vi "CRYOperator Message.vi"() -> ()   [LabVIEW 2013]
uses:
  SubVI/CRYMisc vis settings global.vi
panel:
  in  "sButton":string
  in  "sOperator Type":string
  in  "index":i32
  in  "StateOut":bool
  in  "Stop":bool
  in  "pVI":refnum<vi>
  in  "sMsgCommand":string="REMOTE_COMMAND"
  # "Operator Message Processing."
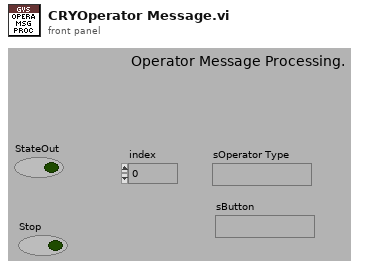
[diagram p1: front panel]
types:
  T1 = cluster{"VI Ref":refnum<vi>[], "VI nID":i32[], "Title nID":i32[]}
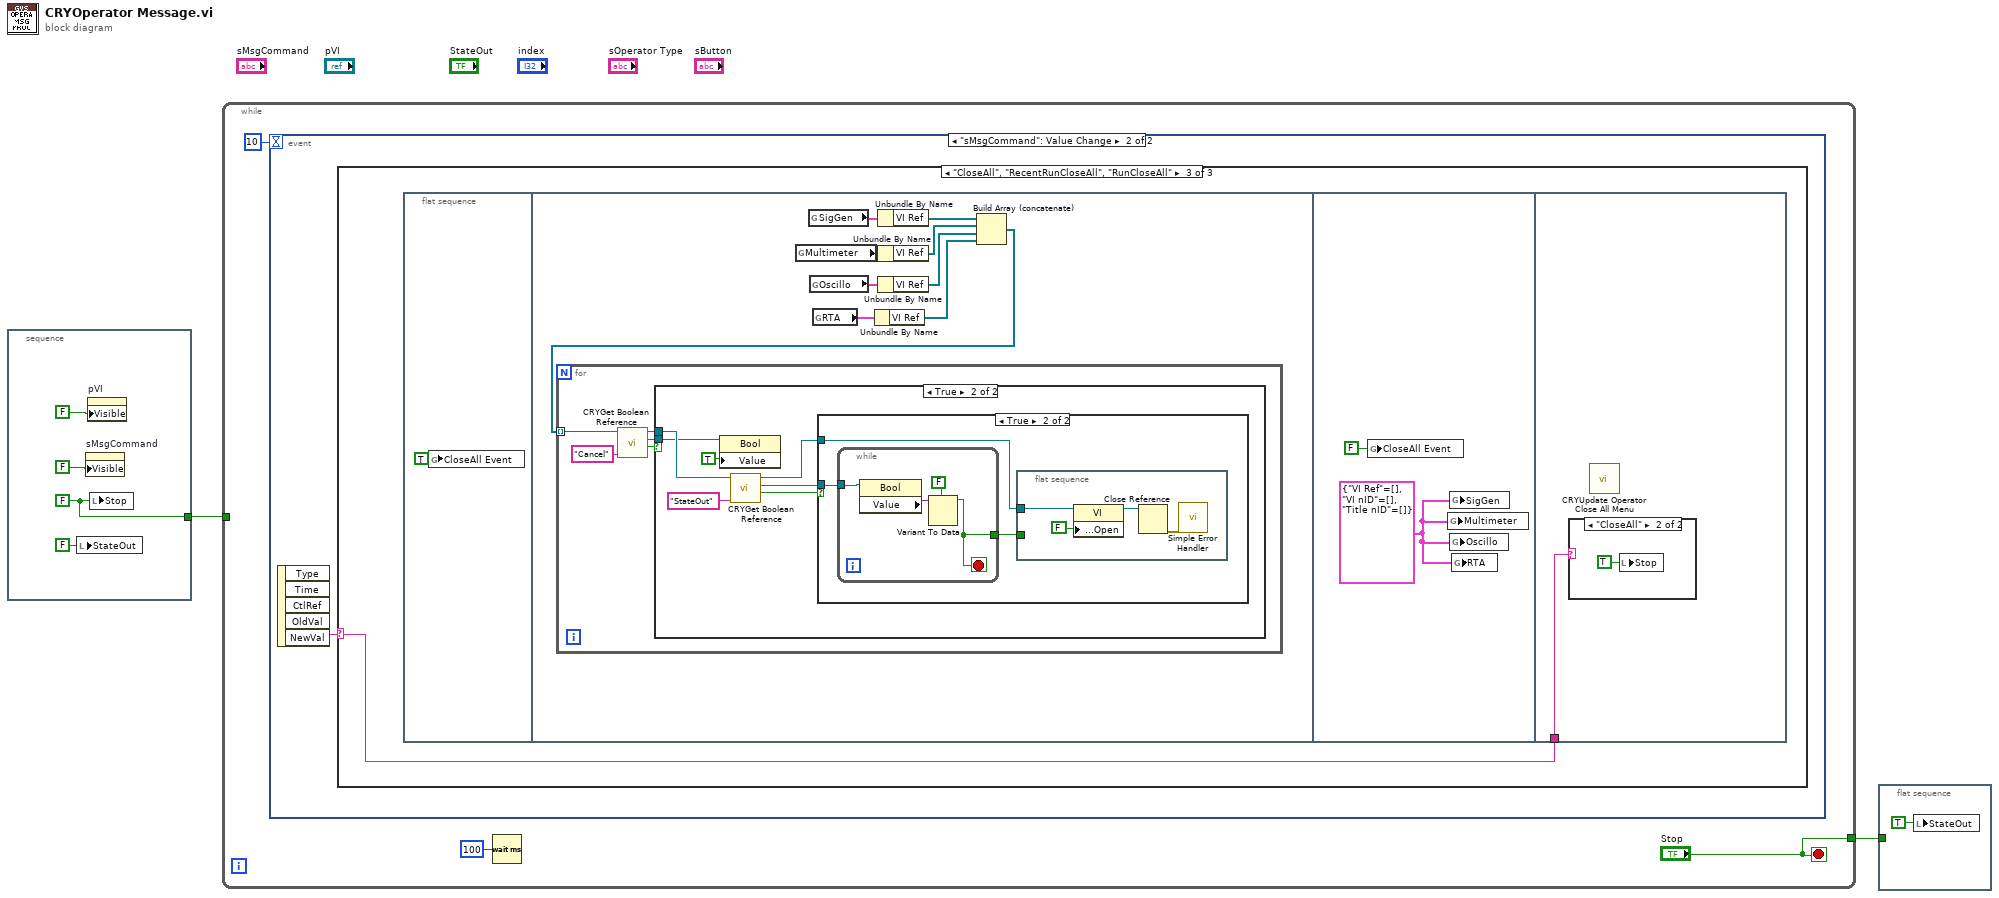
[diagram p0: block diagram]
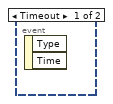
[diagram p2: hidden frame]
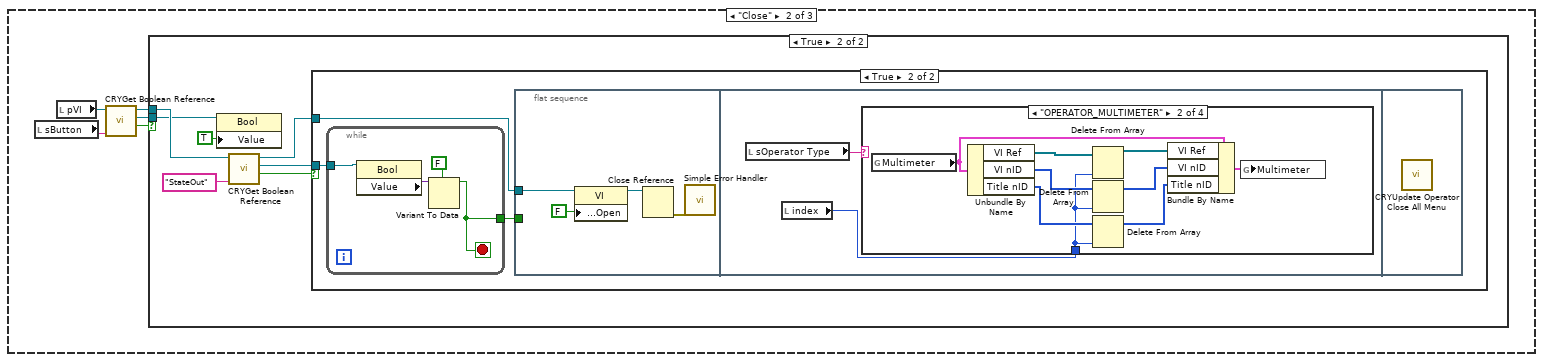
[diagram p4: hidden frame]
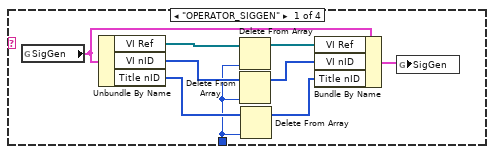
[diagram p7: hidden frame]
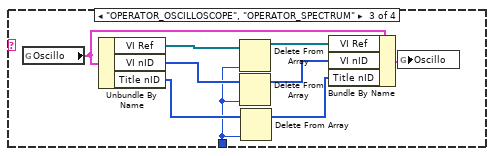
[diagram p8: hidden frame]
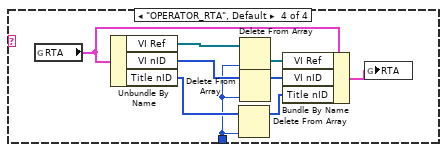
[diagram p9: hidden frame]
diagram:
  n1 = stacked-sequence {
    tunnel: [w3] -> w1
    frame #0 {
      w3 = FALSE ("bStop")
      n2 = local write "StateOut"(FALSE ("StateOut")) -> ()
      n3 = property on="sMsgCommand" class="Str"("Visible"=FALSE) -> ()  [unwired: 2 in, 2 out]
      n4 = property on="pVI" class="VIRef (strict)"("Visible"=FALSE) -> ()  [unwired: 2 in, 2 out]
      n5 = local write "Stop"(w3) -> ()
    }
  }
  n6 = while {
    tunnel: ["Stop"] -> w2
    tunnel: w1 -> [_]
    stop <- "Stop" stop-if-true
    n7 = event shown="[1] \"sMsgCommand\": Value Change" {
      selector: _ -> [_ _]
      dyn-events: _ -> [_ _]
      timeout: 10 -> [_ _]
      event Timeout {
        n8 = event-data() -> ()  [unwired: 3 out]
      }
      event "sMsgCommand": Value Change {
        n9 = event-data() -> ("NewVal"=w10:string)  [unwired: 5 out]
        n10 = case shown="\"CloseAll\", \"RecentRunCloseAll\", \"RunCloseAll\"" w10 {
          selector: w10 -> [_ _ w72]
          frame Default {
          }
          frame "Close" {
            n11 = local read "sButton"() -> (w11:string)
            n12 = local read "pVI"() -> (w12:refnum<vi>)
            n13 = call "CRYGet Boolean Reference.vi"("Label Name"=w11, "VI Refnum"=w12) -> ("Exist?"=w15:bool, "Boolean Ref"=w13:refnum<vi>, "VI Refnum Out"=w14:refnum<vi>)  [unwired: 7 in]
            n14 = case shown="True" w15 {
              tunnel: w14 -> [_ w18]
              tunnel: w13 -> [_ w17]
              frame False {
              }
              frame True {
                n15 = property class="Bool"(reference=w17, "Value"=TRUE ("Boolean")) -> ()  [unwired: 1 in, 2 out]
                n16 = call "CRYGet Boolean Reference.vi"("Label Name"="StateOut", "VI Refnum"=w18) -> ("Exist?"=w22:bool, "Boolean Ref"=w21:refnum<vi>, "VI Refnum Out"=w20:refnum<vi>)  [unwired: 7 in]
                n17 = case shown="True" w22 {
                  tunnel: w21 -> [_ w25]
                  tunnel: w20 -> [_ w23]
                  frame False {
                  }
                  frame True {
                    n18 = while {
                      tunnel: w25 -> [w71]
                      tunnel: [w68] -> w24
                      stop <- w68 stop-if-true
                      n19 = property class="Bool"(reference=w71) -> ("Value"=w70:variant)  [unwired: 1 in, 2 out]
                      n20 = Variant To Data(type=FALSE ("Boolean"), Variant=w70) -> (data=w68:bool)  [unwired: 1 in, 1 out]
                    }
                    n21 = flat-sequence {
                      tunnel: w23 -> [w29]
                      tunnel: w24 -> [_]
                      frame #0 {
                        n22 = property class="VI"(reference=w29, "Front Panel.Open"=FALSE ("Front Panel Window:Open")) -> (reference out=w28:refnum<vi>)  [unwired: 1 in, 1 out]
                        n23 = Close Reference(reference=w28) -> (error out=w26:errorcluster)  [unwired: 1 in]
                        n24 = call <vilib>:"Simple Error Handler.vi"("error in (no error)"=w26) -> ()  [unwired: 2 in, 7 out]
                      }
                      frame #1 {
                        n25 = local read "sOperator Type"() -> (w31:string)
                        n26 = local read "index"() -> (w30:i32)
                        n27 = case shown="\"OPERATOR_MULTIMETER\"" w31 {
                          tunnel: w30 -> [w33 w41 w50 w60]
                          frame "OPERATOR_SIGGEN" {
                            n28 = global read "CRYMisc vis settings global.vi" "SigGen"() -> (w35:T1)
                            n29 = Unbundle By Name(w35) -> ("VI Ref"=w37:refnum<vi>[], "VI nID"=w38:i32[], "Title nID"=w34:i32[])
                            n30 = Delete From Array(array=w37, index=w33) -> (array with subset deleted=w39:refnum<vi>[])  [unwired: 1 in, 1 out]
                            n31 = Delete From Array(array=w38, index=w33) -> (array with subset deleted=w40:i32[])  [unwired: 1 in, 1 out]
                            n32 = Delete From Array(array=w34, index=w33) -> (array with subset deleted=w32:i32[])  [unwired: 1 in, 1 out]
                            n33 = Bundle By Name(cluster=w35, "VI Ref"=w39, "VI nID"=w40, "Title nID"=w32) -> (w36:T1)
                            n34 = global write "CRYMisc vis settings global.vi" "SigGen"(w36) -> ()
                          }
                          frame "OPERATOR_MULTIMETER" {
                            n35 = global read "CRYMisc vis settings global.vi" "Multimeter"() -> (w44:T1)
                            n36 = Unbundle By Name(w44) -> ("VI Ref"=w46:refnum<vi>[], "VI nID"=w47:i32[], "Title nID"=w43:i32[])
                            n37 = Delete From Array(array=w46, index=w41) -> (array with subset deleted=w48:refnum<vi>[])  [unwired: 1 in, 1 out]
                            n38 = Delete From Array(array=w47, index=w41) -> (array with subset deleted=w49:i32[])  [unwired: 1 in, 1 out]
                            n39 = Delete From Array(array=w43, index=w41) -> (array with subset deleted=w42:i32[])  [unwired: 1 in, 1 out]
                            n40 = Bundle By Name(cluster=w44, "VI Ref"=w48, "VI nID"=w49, "Title nID"=w42) -> (w45:T1)
                            n41 = global write "CRYMisc vis settings global.vi" "Multimeter"(w45) -> ()
                          }
                          frame "OPERATOR_OSCILLOSCOPE", "OPERATOR_SPECTRUM" {
                            n42 = global read "CRYMisc vis settings global.vi" "Oscillo"() -> (w53:T1)
                            n43 = Unbundle By Name(w53) -> ("VI Ref"=w55:refnum<vi>[], "VI nID"=w56:i32[], "Title nID"=w52:i32[])
                            n44 = Delete From Array(array=w55, index=w50) -> (array with subset deleted=w57:refnum<vi>[])  [unwired: 1 in, 1 out]
                            n45 = Delete From Array(array=w56, index=w50) -> (array with subset deleted=w58:i32[])  [unwired: 1 in, 1 out]
                            n46 = Delete From Array(array=w52, index=w50) -> (array with subset deleted=w51:i32[])  [unwired: 1 in, 1 out]
                            n47 = Bundle By Name(cluster=w53, "VI Ref"=w57, "VI nID"=w58, "Title nID"=w51) -> (w54:T1)
                            n48 = global write "CRYMisc vis settings global.vi" "Oscillo"(w54) -> ()
                          }
                          frame "OPERATOR_RTA", Default {
                            n49 = global read "CRYMisc vis settings global.vi" "RTA"() -> (w62:T1)
                            n50 = Unbundle By Name(w62) -> ("VI Ref"=w64:refnum<vi>[], "VI nID"=w65:i32[], "Title nID"=w61:i32[])
                            n51 = Delete From Array(array=w61, index=w60) -> (array with subset deleted=w59:i32[])  [unwired: 1 in, 1 out]
                            n52 = Delete From Array(array=w64, index=w60) -> (array with subset deleted=w66:refnum<vi>[])  [unwired: 1 in, 1 out]
                            n53 = Delete From Array(array=w65, index=w60) -> (array with subset deleted=w67:i32[])  [unwired: 1 in, 1 out]
                            n54 = Bundle By Name(cluster=w62, "VI Ref"=w66, "VI nID"=w67, "Title nID"=w59) -> (w63:T1)
                            n55 = global write "CRYMisc vis settings global.vi" "RTA"(w63) -> ()
                          }
                        }
                      }
                      frame #2 {
                        n56 = call "CRYUpdate Operator Close All Menu.vi"() -> ()  [unwired: 12 in]
                      }
                    }
                  }
                }
              }
            }
          }
          frame "CloseAll", "RecentRunCloseAll", "RunCloseAll" {
            n57 = flat-sequence {
              tunnel: w72 -> [w108]
              frame #0 {
                n58 = global write "CRYMisc vis settings global.vi" "CloseAll Event"(TRUE ("CloseAll Event")) -> ()
              }
              frame #1 {
                n59 = global read "CRYMisc vis settings global.vi" "Multimeter"() -> (w81:T1)
                n60 = global read "CRYMisc vis settings global.vi" "SigGen"() -> (w82:T1)
                n61 = global read "CRYMisc vis settings global.vi" "Oscillo"() -> (w80:T1)
                n62 = global read "CRYMisc vis settings global.vi" "RTA"() -> (w79:T1)
                n63 = Unbundle By Name(w79) -> ("VI Ref"=w75:refnum<vi>[])
                n64 = Unbundle By Name(w82) -> ("VI Ref"=w78:refnum<vi>[])
                n65 = Unbundle By Name(w81) -> ("VI Ref"=w77:refnum<vi>[])
                n66 = Unbundle By Name(w80) -> ("VI Ref"=w76:refnum<vi>[])
                n67 = Build Array (concatenate)(w78, w77, w76, w75) -> (w74:refnum<vi>[])
                n68 = for {
                  tunnel: w74 -> [w86] mode=indexing
                  n69 = call "CRYGet Boolean Reference.vi"("Label Name"="Cancel", "VI Refnum"=w86) -> ("Exist?"=w85:bool, "Boolean Ref"=w83:refnum<vi>, "VI Refnum Out"=w84:refnum<vi>)  [unwired: 7 in]
                  n70 = case shown="True" w85 {
                    tunnel: w84 -> [_ w90]
                    tunnel: w83 -> [_ w89]
                    frame False {
                    }
                    frame True {
                      n71 = property class="Bool"(reference=w89, "Value"=TRUE ("Boolean")) -> ()  [unwired: 1 in, 2 out]
                      n72 = call "CRYGet Boolean Reference.vi"("Label Name"="StateOut", "VI Refnum"=w90) -> ("Exist?"=w94:bool, "Boolean Ref"=w93:refnum<vi>, "VI Refnum Out"=w92:refnum<vi>)  [unwired: 7 in]
                      n73 = case shown="True" w94 {
                        tunnel: w93 -> [_ w97]
                        tunnel: w92 -> [_ w95]
                        frame False {
                        }
                        frame True {
                          n74 = while {
                            tunnel: w97 -> [w105]
                            tunnel: [w102] -> w96
                            stop <- w102 stop-if-true
                            n75 = property class="Bool"(reference=w105) -> ("Value"=w104:variant)  [unwired: 1 in, 2 out]
                            n76 = Variant To Data(type=FALSE ("Boolean"), Variant=w104) -> (data=w102:bool)  [unwired: 1 in, 1 out]
                          }
                          n77 = flat-sequence {
                            tunnel: w95 -> [w101]
                            tunnel: w96 -> [_]
                            frame #0 {
                              n78 = property class="VI"(reference=w101, "Front Panel.Open"=FALSE ("Front Panel Window:Open")) -> (reference out=w100:refnum<vi>)  [unwired: 1 in, 1 out]
                              n79 = Close Reference(reference=w100) -> (error out=w98:errorcluster)  [unwired: 1 in]
                              n80 = call <vilib>:"Simple Error Handler.vi"("error in (no error)"=w98) -> ()  [unwired: 2 in, 7 out]
                            }
                          }
                        }
                      }
                    }
                  }
                }
              }
              frame #2 {
                w106 = T1 {"VI Ref"=[], "VI nID"=[], "Title nID"=[]} ("RTA")
                n81 = global write "CRYMisc vis settings global.vi" "CloseAll Event"(FALSE ("CloseAll Event")) -> ()
                n82 = global write "CRYMisc vis settings global.vi" "Multimeter"(w106) -> ()
                n83 = global write "CRYMisc vis settings global.vi" "SigGen"(w106) -> ()
                n84 = global write "CRYMisc vis settings global.vi" "Oscillo"(w106) -> ()
                n85 = global write "CRYMisc vis settings global.vi" "RTA"(w106) -> ()
              }
              frame #3 {
                n86 = case shown="\"CloseAll\"" w108 {
                  frame "False", Default {
                  }
                  frame "CloseAll" {
                    n87 = local write "Stop"(TRUE ("Stop")) -> ()
                  }
                }
                n88 = call "CRYUpdate Operator Close All Menu.vi"() -> ()  [unwired: 12 in]
              }
            }
          }
        }
      }
    }
    n89 = Wait (ms)(milliseconds to wait=u32 100) -> ()  [unwired: 1 out]
  }
  n90 = flat-sequence {
    tunnel: w2 -> [_]
    frame #0 {
      n91 = local write "StateOut"(TRUE ("StateOut")) -> ()
    }
  }
